vi "Untitled 8.vi"() -> ()   [LabVIEW 2021]
panel:
  out "Boolean":bool
  out "concatenated string":string
  in  "Times":dbl[](array[numeric])
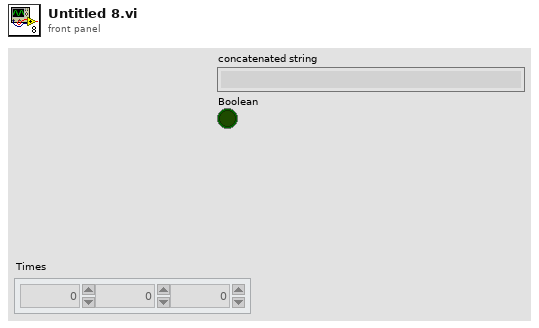
[diagram p1: front panel]
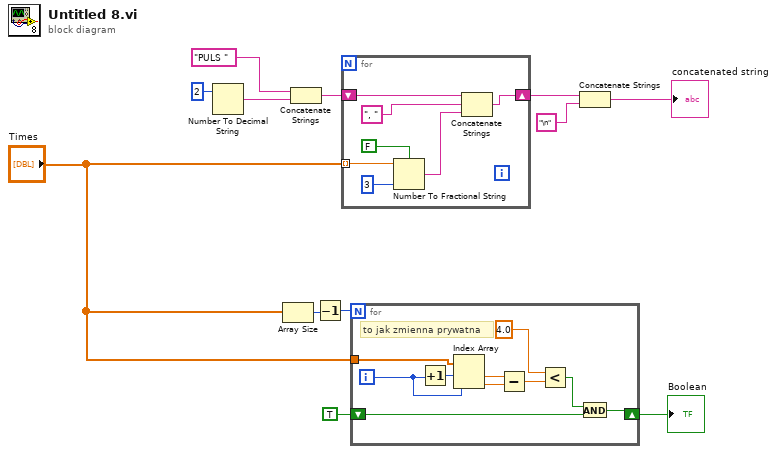
[diagram p0: block diagram]
diagram:
  n1 = Number To Decimal String(number=2) -> (decimal integer string=w11:string)  [unwired: 1 in]
  n2 = Array Size(array="Times") -> (size(s)=w5:i32)
  n3 = Concatenate Strings("PULS " ("string"), w11) -> (w9:string)
  n4 = Decrement(x=w5) -> (x-1=w4:i32)
  n5 = for {
    tunnel: "Times" -> [w17] mode=indexing
    shift-right: [w19] -> w8
    shift-left: w9 -> [w18]
    n6 = Number To Fractional String(use system decimal point (T)=FALSE, number=w17, precision (6)=i16 3) -> (F-format string=w14:string)  [unwired: 1 in]
    n7 = Concatenate Strings(w18, ", " ("string"), w14) -> (w19:string)
  }
  n8 = for {
    N: w4 -> [_]
    tunnel: "Times" -> [w26]
    shift-right: [w21] -> w1
    shift-left: TRUE -> [w25]
    i -> [w20]
    # "to jak zmienna prywatna"
    n9 = Increment(x=w20) -> (x+1=w29:i32)
    n10 = Index Array(array=w26, index #1=w29, index #2=w20) -> (element #1=w28:dbl, element #2=w27:dbl)
    n11 = Subtract(x=w28, y=w27) -> (x-y=w24:dbl)
    n12 = Less?(x=4.0, y=w24) -> (x < y?=w22:bool)
    n13 = And(x=w22, y=w25) -> (x .and. y?=w21:bool)
  }
  "Boolean" <- w1
  n14 = Concatenate Strings(w8, "\n" ("string")) -> (→"concatenated string":string)
